vi "Talker.vi"(0 "Add in":refnum<class "Add.lvclass">, 5 "Subpanel Ref":refnum<vi>, 11 "Error In":errorcluster) -> (4 "Add out":refnum<class "Add.lvclass">, 15 "Error Out":errorcluster)   [LabVIEW 2020, in "Add.lvclass"]
doc: "Method to call the UI Method. This will pass the object to the UI Method which will do the operation and return the object to the main vi."
uses:
  Add.lvclass
  D:/Github Projects/LV_Assignment/Tasks/A18/A18/Classes/Arithmetic_Operations/Arithmetic_Operations.lvclass
  UI.vi
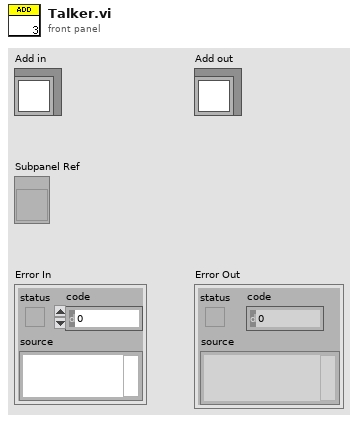
[diagram p1: front panel]
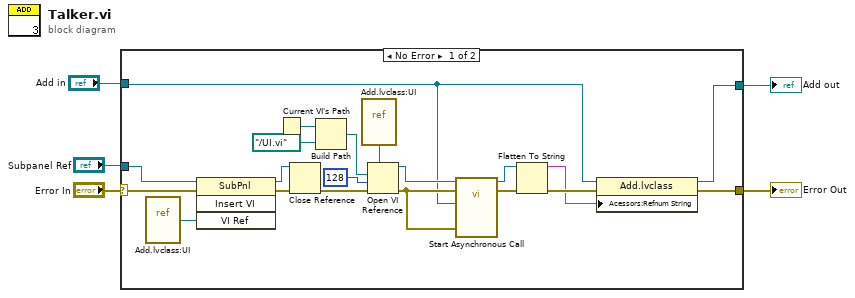
[diagram p0: block diagram]
diagram:
  n1 = case shown="No Error" "Error In" {
    selector: "Error In" -> [w22 w27]
    tunnel: [w11 w27] -> w4
    tunnel: [w10 w26] -> w2
    tunnel: "Add in" -> [w9 w26]
    tunnel: "Subpanel Ref" -> [w21 _]
    frame No Error {
      n2 = vi-ref "Add.lvclass:UI.vi"() -> (w12:refnum<vi>)
      n3 = invoke on="Invoke Node" class="SubPnl" method="Insert VI"(reference=w21, error in=w22, "VI Ref"=w12) -> (reference out=w13:refnum<vi>, error out=w14:errorcluster)  [unwired: 1 in, 2 out]
      n4 = Current VI's Path() -> (path=w16:path)
      n5 = Close Reference(reference=w13, error in (no error)=w14) -> (error out=w18:errorcluster)
      n6 = Build Path(base path=w16, name or relative path=path "../UI.vi") -> (appended path=w19:path)
      n7 = vi-ref "Add.lvclass:UI.vi"() -> (w17:refnum<vi>)
      n8 = Open VI Reference(type specifier VI Refnum (for type only)=w17, vi path=w19, options=128, error in (no error)=w18) -> (vi reference=w20:refnum<vi>, error out=w25:errorcluster)  [unwired: 2 in]
      n9 = call-by-ref "Start Asynchronous Call"(reference=w20, error in=w25, "Add.lvclass"=w9, "Error In"=w25) -> (reference out=w7:refnum<vi>, error out=w24:errorcluster)  [unwired: 11 in, 3 out]
      n10 = Flatten To String(anything=w7, error in (no error)=w24) -> (data string=w6:string, error out=w8:errorcluster)  [unwired: 2 in, 1 out]
      n11 = property class="Add.lvclass"(reference=w9, error in=w8, "Acessors:Refnum String"=w6) -> (reference out=w10:refnum<class "Add.lvclass">, error out=w11:errorcluster)
    }
    frame Error {
    }
  }
  "Error Out" <- w4
  "Add out" <- w2
